vi "Разбрка кластра.vi"() -> ()   [LabVIEW 2017]
panel:
  out "Boolean":bool
  out "Numeric":dbl
  out "String":string
  in  "Cluster":T1
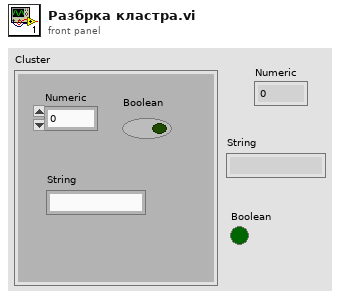
[diagram p1: front panel]
types:
  T1 = cluster{"Numeric":dbl, "Boolean":bool, "String":string}
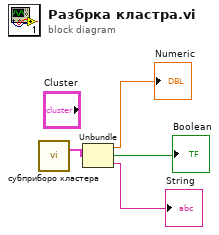
[diagram p0: block diagram]
diagram:
  n1 = call "субприборо кластера.vi"() -> ("Cluster"=w1:T1)  [unwired: 11 in]
  n2 = Unbundle(w1) -> ("Numeric"=→"Numeric":dbl, "Boolean"=→"Boolean":bool, "String"=→"String":string)
